vi "11_random number from 0 to 99.vi"() -> ()   [LabVIEW 2018]
panel:
  out "Numeric Integer":i64
  # "Develop HMI (Human Machine Interface) to display random number from 0 to 99\nusing while loop for only 5 times and timer 2.5 mili sec"
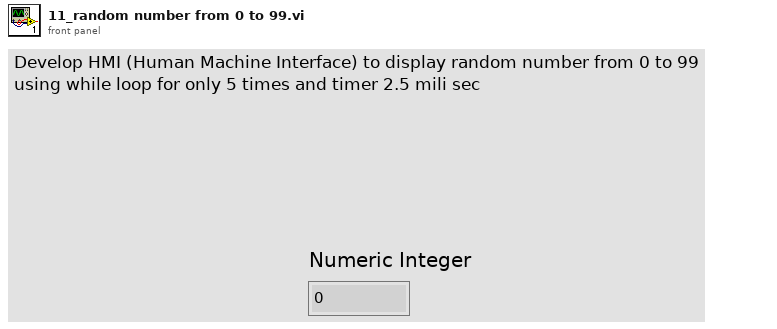
[diagram p1: front panel]
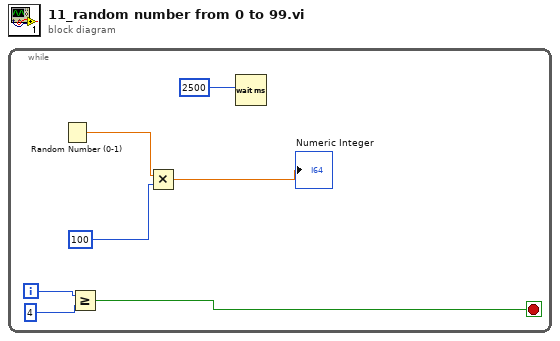
[diagram p0: block diagram]
diagram:
  n1 = while {
    i -> [w3]
    stop <- w1 stop-if-true
    n2 = Random Number (0-1)() -> (number: 0 to 1=w7:dbl)
    n3 = Greater Or Equal?(x=w3, y=4) -> (x >= y?=w1:bool)
    n4 = Multiply(x=w7, y=100) -> (x*y=→"Numeric Integer":dbl)
    n5 = Wait (ms)(milliseconds to wait=u32 2500 ("millisecond timer value")) -> ()  [unwired: 1 out]
  }
